vi "StartUp Sequence Open Loop Rev 1.4.vi"() -> ()   [LabVIEW 2017]
panel:
  in  "Set Pump Value 1":string
  out "Pump Value 2":string
  in  "Soft Shut Off":bool
  out "Pump Value 1":string
  in  "Send Pump":bool
  in  "Send Command":bool
  in  "Custom Command":string
  out "Startup Success":bool
  in  "Output File":path
  in  "Shut Off":bool
  out "ECU COM Port Out":refnum<visa-resource-name>
  out "Throttle Position":string
  out "Turbine RPM":string
  out "Turbine Temp":string
  out "Error Out":errorcluster
  in  "Error In":errorcluster
  in  "ECU COM Port":refnum<visa-resource-name>
  out "Turbine State":string
  in  "Strt Sqnc":bool
  # "Note: save to a .csv file"
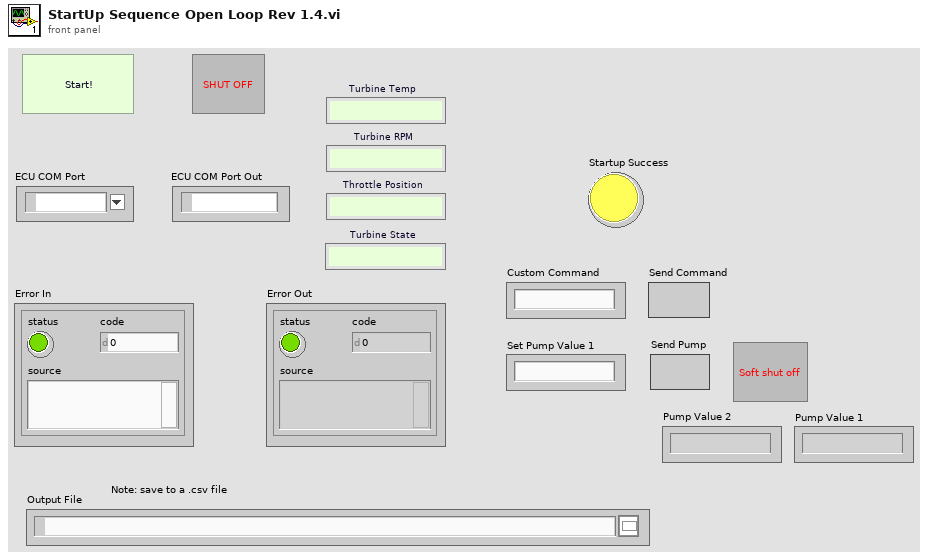
[diagram p1: front panel]
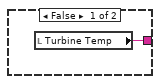
[diagram p4: hidden frame]
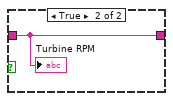
[diagram p5: hidden frame]
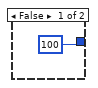
[diagram p7: hidden frame]
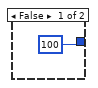
[diagram p8: hidden frame]
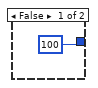
[diagram p9: hidden frame]
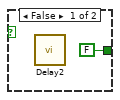
[diagram p11: hidden frame]
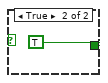
[diagram p12: hidden frame]
diagram:
  w7 = 21 ("Pulse Width")
  w8 = 160 ("Voltage")
  w13 = 16 ("Pulse Width")
  w14 = 160 ("Voltage")
  w4 = 255 ("y")
  w5 = 80 ("y")
  # "Disengage Starter Motor"
  # "Starter Motor 55%"
  # "Start button is inside a while loop that doesn't progess until True"
  # "Fuel Pump Mode 2"
  # "GlowPlugOff"
  # "Start Up\nFuelPumpMode 1"
  # "BurnerValveIgnitionPercent"
  # "If False, each Case structure is set\nto an arbitrary Delay time of 0.2 s"
  # "Each Stage is inside a while loop so that \nthe sequence doesn't progress until True"
  n1 = call "Initialize Com Port.vi"("Error In"="Error In", "ECU COM Port"="ECU COM Port") -> ("Error Out"=w28:errorcluster, "ECU COM Port Out"=w27:refnum<visa-resource-name>)  [unwired: 8 in]
  n2 = while {
    tunnel: w28 -> [w125]
    tunnel: [w125] -> w26
    stop <- "Strt Sqnc" stop-if-true
  }
  n3 = call "Initialize Output File.vi"("error in (no error)"=w26, "File Path Control"="Output File") -> ("error out"=w3:errorcluster)  [unwired: 9 in]
  n4 = flat-sequence {
    tunnel: w3 -> [w127]
    tunnel: [w127] -> w18
    frame #0 {
      n5 = local write "Strt Sqnc"(FALSE ("Strt Sqnc")) -> ()
    }
  }
  n6 = flat-sequence {
    tunnel: [w130] -> w2
    tunnel: w3 -> [w130]
    frame #0 {
      w129 = "0" ("Pump Value 1")
      n7 = local write "Pump Value 2"(w129) -> ()
      n8 = local write "Pump Value 1"(w129) -> ()
    }
  }
  n9 = while {
    tunnel: w2 -> [w148]
    tunnel: w27 -> [w147]
    tunnel: "Output File" -> [w144]
    stop <- w143 continue-if-true
    n10 = call "Get Engine Update.vi"("Error In"=w148, "ECU COM Port"=w147) -> ("Error Out"=w145:errorcluster, "Temperature"=w136:string, "RPMs"=w140:string, "ECU COM Port Out"=w142:refnum<visa-resource-name>)  [unwired: 6 in]
    n11 = call "Time Delay4"() -> ()  [unwired: 11 in, 1 out]
    n12 = call "Safety Check.vi"("Temperature"=w136, "RPMs"=w140) -> ("Safe?"=w143:bool)  [unwired: 9 in]
    n13 = Not Equal?(x=w140, y="") -> (x != y?=w138:bool)
    n14 = Not Equal?(x=w136, y="") -> (x != y?=w135:bool)
    n15 = case shown="False" w143 {
      selector: w143 -> [w153 w155]
      tunnel: w142 -> [w154 _]
      tunnel: [w153 w155] -> w141
      frame False {
        n16 = call "Emergency Shutoff.vi"("ECU COM Port"=w154) -> ()  [unwired: 9 in, 2 out]
      }
      frame True {
      }
    }
    n17 = case shown="False" w138 {
      tunnel: w140 -> [_ w152]
      tunnel: [w151 w152] -> w133
      frame False {
        n18 = local read "Turbine RPM"() -> (w151:string)
      }
      frame True {
        "Turbine RPM" <- w152
      }
    }
    n19 = case shown="True" w135 {
      tunnel: w136 -> [_ w150]
      tunnel: [w149 w150] -> w134
      frame False {
        n20 = local read "Turbine Temp"() -> (w149:string)
      }
      frame True {
        "Turbine Temp" <- w150
      }
    }
    n21 = Not(x=w141) -> (.not. x?=w146:bool)
    n22 = Stop(stop? (T)=w146) -> ()
    n23 = local read "Pump Value 2"() -> (w131:string)
    n24 = local read "Pump Value 1"() -> (w132:string)
    n25 = call "Write Data to Output File.vi"("Pump Value 2"=w131, "Pump Value 1"=w132, "Error In"=w145, "Temperature"=w134, "RPM"=w133, "File Path Control"=w144) -> ()  [unwired: 5 in, 1 out]
  }
  n26 = while {
    tunnel: w27 -> [w157]
    tunnel: w28 -> [_]
    stop <- FALSE stop-if-true
    n27 = case shown="True" "Send Command" {
      tunnel: "Custom Command" -> [_ w161]
      tunnel: w157 -> [_ w160]
      frame False {
      }
      frame True {
        n28 = call "Time Delay3"() -> ()  [unwired: 11 in, 1 out]
        n29 = VISA Write(VISA resource name=w160, write buffer=w161) -> ()  [unwired: 1 in, 3 out]
      }
    }
  }
  n30 = flat-sequence {
    tunnel: w18 -> [_]
    frame #0 {
      n31 = local write "Turbine State"("Initializing Motor") -> ()
    }
  }
  n32 = while {
    tunnel: ["Shut Off"] -> w122
    tunnel: "ECU COM Port" -> [w163]
    stop <- "Shut Off" stop-if-true
    # "Turns off each individual component"
    n33 = case shown="True" "Shut Off" {
      tunnel: w163 -> [_ w167]
      frame False {
      }
      frame True {
        n34 = call "Emergency Shutoff.vi"("ECU COM Port"=w167) -> ("Error Out"=w166:errorcluster)  [unwired: 9 in, 1 out]
        n35 = local write "Output File"(path "" ("Output File")) -> ()
        n36 = flat-sequence {
          tunnel: w166 -> [w168]
          tunnel: [w168] -> _
          frame #0 {
            n37 = local write "Strt Sqnc"(FALSE ("Strt Sqnc")) -> ()
          }
        }
      }
    }
  }
  n38 = call "Set Glow Plug Duty Cycle.vi"("Error In"=w18, "Duty Cycle"=6, "ECU COM Port"=w27) -> ("Error Out"=w113:errorcluster, "ECU COM Port Out"=w110:refnum<visa-resource-name>)  [unwired: 7 in]
  n39 = call "Delay"("error in (no error)"=w113) -> ("error out"=w112:errorcluster)  [unwired: 10 in]
  n40 = call "Set Glow Plug Duty Cycle.vi"("Error In"=w112, "Duty Cycle"=19, "ECU COM Port"=w110) -> ("Error Out"=w111:errorcluster, "ECU COM Port Out"=w106:refnum<visa-resource-name>)  [unwired: 7 in]
  n41 = call "Delay"("error in (no error)"=w111) -> ("error out"=w107:errorcluster)  [unwired: 10 in]
  n42 = call "Set Starter Motor Duty Cycle.vi"("Error In"=w107, "Duty Cycle"=6, "ECU COM Port"=w106) -> ("Error Out"=w105:errorcluster, "ECU COM Port Out"=w103:refnum<visa-resource-name>)  [unwired: 7 in]
  n43 = call "Set Glow Plug Duty Cycle.vi"("Error In"=w105, "Duty Cycle"=15, "ECU COM Port"=w103) -> ("Error Out"=w104:errorcluster, "ECU COM Port Out"=w99:refnum<visa-resource-name>)  [unwired: 7 in]
  n44 = call "Delay"("error in (no error)"=w104) -> ("error out"=w101:errorcluster)  [unwired: 10 in]
  n45 = call "Set Starter Motor Duty Cycle.vi"("Error In"=w101, "Duty Cycle"=4, "ECU COM Port"=w99) -> ("Error Out"=w100:errorcluster, "ECU COM Port Out"=w98:refnum<visa-resource-name>)  [unwired: 7 in]
  n46 = call "Delay"("error in (no error)"=w100) -> ("error out"=w123:errorcluster)  [unwired: 10 in]
  n47 = Stop(stop? (T)=w122) -> ()
  n48 = while {
    tunnel: w123 -> [w172]
    tunnel: w98 -> [w171]
    tunnel: [w171] -> w16
    tunnel: [w172] -> w124
    stop <- w175 stop-if-true
    n49 = local read "Turbine RPM"() -> (w170:string)
    n50 = Decimal String To Number(string=w170) -> (number=w174:i32)  [unwired: 2 in, 1 out]
    n51 = Greater Or Equal?(x=w174, y=3300) -> (x >= y?=w176:bool)
    n52 = case shown="True" w176 {
      tunnel: [FALSE TRUE] -> w175
      frame False {
        n53 = call "Delay2"() -> ()  [unwired: 11 in, 1 out]
      }
      frame True {
      }
    }
  }
  n54 = flat-sequence {
    tunnel: w123 -> [_]
    frame #0 {
      n55 = local write "Turbine State"("Stage1 Check RPM") -> ()
    }
  }
  n56 = call "CmdSeparator7"("error in (no error)"=w124) -> ("error out"=w12:errorcluster)  [unwired: 10 in]
  n57 = call "Set Pump Fow Rate.vi"("Error In"=w12, "Pulse Width"=w13, "Voltage"=w14, "ECU COM Port"=w16) -> ("Error Out"=w17:errorcluster, "ECU COM Port Out"=w15:refnum<visa-resource-name>)  [unwired: 6 in]
  n58 = flat-sequence {
    tunnel: w14 -> [w181]
    tunnel: w13 -> [w180]
    tunnel: w12 -> [_]
    frame #0 {
      n59 = Number To Decimal String(number=w180) -> (decimal integer string=w182:string)  [unwired: 1 in]
      n60 = Number To Decimal String(number=w181) -> (decimal integer string=w183:string)  [unwired: 1 in]
      n61 = local write "Pump Value 2"(w182) -> ()
      n62 = local write "Pump Value 1"(w183) -> ()
    }
  }
  n63 = call "CmdSeparator2"("error in (no error)"=w17) -> ("error out"=w97:errorcluster)  [unwired: 10 in]
  n64 = call "Set Burner Valve Percent.vi"("Error In"=w97, "Percent"=10, "ECU COM Port"=w15) -> ("Error Out"=w96:errorcluster, "ECU COM Port Out"=w86:refnum<visa-resource-name>)  [unwired: 7 in]
  n65 = call "CmdSeparator"("error in (no error)"=w96) -> ("error out"=w95:errorcluster)  [unwired: 10 in]
  n66 = call "Set Burner Valve Percent.vi"("Error In"=w95, "Percent"=31, "ECU COM Port"=w86) -> ("Error Out"=w94:errorcluster, "ECU COM Port Out"=w85:refnum<visa-resource-name>)  [unwired: 7 in]
  n67 = call "CmdSeparator10"("error in (no error)"=w94) -> ("error out"=w93:errorcluster)  [unwired: 10 in]
  n68 = call "Set Burner Valve Percent.vi"("Error In"=w93, "Percent"=35, "ECU COM Port"=w85) -> ("Error Out"=w92:errorcluster, "ECU COM Port Out"=w84:refnum<visa-resource-name>)  [unwired: 7 in]
  n69 = call "CmdSeparator11"("error in (no error)"=w92) -> ("error out"=w91:errorcluster)  [unwired: 10 in]
  n70 = call "Set Burner Valve Percent.vi"("Error In"=w91, "Percent"=39, "ECU COM Port"=w84) -> ("Error Out"=w90:errorcluster, "ECU COM Port Out"=w83:refnum<visa-resource-name>)  [unwired: 7 in]
  n71 = call "CmdSeparator12"("error in (no error)"=w90) -> ("error out"=w89:errorcluster)  [unwired: 10 in]
  n72 = call "Set Burner Valve Percent.vi"("Error In"=w89, "Percent"=43, "ECU COM Port"=w83) -> ("Error Out"=w88:errorcluster, "ECU COM Port Out"=w82:refnum<visa-resource-name>)  [unwired: 7 in]
  n73 = call "CmdSeparator13"("error in (no error)"=w88) -> ("error out"=w87:errorcluster)  [unwired: 10 in]
  n74 = call "Set Burner Valve Percent.vi"("Error In"=w87, "Percent"=47, "ECU COM Port"=w82) -> ("Error Out"=w65:errorcluster, "ECU COM Port Out"=w64:refnum<visa-resource-name>)  [unwired: 7 in]
  n75 = call "CmdSeparator6"("error in (no error)"=w65) -> ("error out"=w67:errorcluster)  [unwired: 10 in]
  n76 = call "Set Burner Valve Percent.vi"("Error In"=w67, "Percent"=51, "ECU COM Port"=w64) -> ("Error Out"=w60:errorcluster, "ECU COM Port Out"=w61:refnum<visa-resource-name>)  [unwired: 7 in]
  n77 = call "CmdSeparator8"("error in (no error)"=w60) -> ("error out"=w63:errorcluster)  [unwired: 10 in]
  n78 = call "Set Burner Valve Percent.vi"("Error In"=w63, "Percent"=55, "ECU COM Port"=w61) -> ("Error Out"=w56:errorcluster, "ECU COM Port Out"=w57:refnum<visa-resource-name>)  [unwired: 7 in]
  n79 = call "CmdSeparator14"("error in (no error)"=w56) -> ("error out"=w59:errorcluster)  [unwired: 10 in]
  n80 = call "Set Burner Valve Percent.vi"("Error In"=w59, "Percent"=59, "ECU COM Port"=w57) -> ("Error Out"=w55:errorcluster, "ECU COM Port Out"=w54:refnum<visa-resource-name>)  [unwired: 7 in]
  n81 = call "CmdSeparator9"("error in (no error)"=w55) -> ("error out"=w121:errorcluster)  [unwired: 10 in]
  n82 = flat-sequence {
    tunnel: w121 -> [_]
    frame #0 {
      n83 = local write "Turbine State"("Stage2 Check Temp.") -> ()
    }
  }
  n84 = while {
    tunnel: w54 -> [w186]
    tunnel: w121 -> [w187]
    tunnel: [w186] -> w71
    tunnel: [w187] -> w72
    stop <- w190 stop-if-true
    # "Stage2Temp(C)"
    n85 = local read "Turbine Temp"() -> (w185:string)
    n86 = Decimal String To Number(string=w185) -> (number=w188:i32)  [unwired: 2 in, 1 out]
    n87 = Greater Or Equal?(x=w188, y=90) -> (x >= y?=w191:bool)
    n88 = case shown="False" w191 {
      tunnel: [FALSE TRUE] -> w190
      frame False {
        n89 = call "Delay3"() -> ()  [unwired: 11 in, 1 out]
      }
      frame True {
      }
    }
  }
  n90 = call "Set Glow Plug Duty Cycle.vi"("Error In"=w72, "Duty Cycle"=0, "ECU COM Port"=w71) -> ("Error Out"=w70:errorcluster, "ECU COM Port Out"=w9:refnum<visa-resource-name>)  [unwired: 7 in]
  n91 = call "CmdSeparator3"("error in (no error)"=w70) -> ("error out"=w6:errorcluster)  [unwired: 10 in]
  n92 = call "Set Pump Fow Rate.vi"("Error In"=w6, "Pulse Width"=w7, "Voltage"=w8, "ECU COM Port"=w9) -> ("Error Out"=w11:errorcluster, "ECU COM Port Out"=w10:refnum<visa-resource-name>)  [unwired: 6 in]
  n93 = call "Set Burner Valve Percent.vi"("Error In"=w11, "Percent"=80, "ECU COM Port"=w10) -> ("Error Out"=w53:errorcluster, "ECU COM Port Out"=w68:refnum<visa-resource-name>)  [unwired: 7 in]
  n94 = flat-sequence {
    tunnel: w8 -> [w195]
    tunnel: w7 -> [w194]
    tunnel: w6 -> [_]
    frame #0 {
      n95 = Number To Decimal String(number=w194) -> (decimal integer string=w196:string)  [unwired: 1 in]
      n96 = Number To Decimal String(number=w195) -> (decimal integer string=w197:string)  [unwired: 1 in]
      n97 = local write "Pump Value 2"(w196) -> ()
      n98 = local write "Pump Value 1"(w197) -> ()
    }
  }
  n99 = call "CmdSeparator18"("error in (no error)"=w53) -> ("error out"=w52:errorcluster)  [unwired: 10 in]
  n100 = call "Set Fuel Valve Percent.vi"("Error In"=w52, "Percent"=12, "ECU COM Port"=w68) -> ("Error Out"=w51:errorcluster, "ECU COM Port Out"=w69:refnum<visa-resource-name>)  [unwired: 7 in]
  n101 = call "CmdSeparator16"("error in (no error)"=w51) -> ("error out"=w119:errorcluster)  [unwired: 10 in]
  n102 = for {
    N: 4 -> [_]
    tunnel: [w198] -> _
    tunnel: [w212] -> _
    tunnel: w69 -> [w204]
    tunnel: w119 -> [w205]
    shift-right: [w203] -> w47
    shift-left: 12 -> [w209]
    shift-right: [w200] -> _
    shift-left: 80 -> [w206]
    tunnel: [w212] -> w42 mode=indexing
    tunnel: [w198] -> w48 mode=indexing
    n103 = Less?(x=w209, y=100) -> (x < y?=w210:bool)
    n104 = Less?(x=w206, y=100) -> (x < y?=w207:bool)
    n105 = case shown="True" w207 {
      tunnel: w206 -> [_ w216]
      tunnel: [100 w214] -> w200
      frame False {
      }
      frame True {
        n106 = Add(x=w216, y=5) -> (x+y=w214:i32)
      }
    }
    n107 = case shown="True" w210 {
      tunnel: w209 -> [_ w220]
      tunnel: [100 w218] -> w203
      frame False {
      }
      frame True {
        n108 = Add(x=w220, y=6) -> (x+y=w218:i32)
      }
    }
    n109 = call "Set Fuel Valve Percent.vi"("Error In"=w205, "Percent"=w203, "ECU COM Port"=w204) -> ("Error Out"=w202:errorcluster, "ECU COM Port Out"=w199:refnum<visa-resource-name>)  [unwired: 7 in]
    n110 = call "Set Burner Valve Percent.vi"("Error In"=w202, "Percent"=w200, "ECU COM Port"=w199) -> ("Error Out"=w201:errorcluster, "ECU COM Port Out"=w198:refnum<visa-resource-name>)  [unwired: 7 in]
    n111 = call "CmdSeparator17"("error in (no error)"=w201) -> ("error out"=w212:errorcluster)  [unwired: 10 in]
  }
  n112 = flat-sequence {
    tunnel: w42 -> [_]
    frame #0 {
      n113 = local write "Turbine State"("Pump Ramp Up") -> ()
    }
  }
  n114 = for {
    N: 10 -> [_]
    tunnel: [w228] -> w30
    tunnel: [w239] -> w33
    shift-right: [w235] -> _
    shift-left: w47 -> [w236]
    tunnel: w42 -> [w232] mode=indexing
    tunnel: w48 -> [w231] mode=indexing
    shift-right: [w224] -> w44
    shift-left: 21 -> [w225]
    w223 = 160 ("y")
    n115 = Less?(x=w236, y=100) -> (x < y?=w237:bool)
    n116 = Add(x=w225, y=1) -> (x+y=w224:i32)
    n117 = case shown="True" w237 {
      tunnel: w236 -> [_ w247]
      tunnel: [100 w245] -> w235
      frame False {
      }
      frame True {
        n118 = Add(x=w247, y=5) -> (x+y=w245:i32)
      }
    }
    n119 = call "Set Fuel Valve Percent.vi"("Error In"=w232, "Percent"=w235, "ECU COM Port"=w231) -> ("Error Out"=w234:errorcluster, "ECU COM Port Out"=w233:refnum<visa-resource-name>)  [unwired: 7 in]
    n120 = call "Set Burner Valve Percent.vi"("Error In"=w234, "Percent"=100 ("y"), "ECU COM Port"=w233) -> ("Error Out"=w222:errorcluster, "ECU COM Port Out"=w229:refnum<visa-resource-name>)  [unwired: 7 in]
    n121 = call "Set Pump Fow Rate.vi"("Error In"=w222, "Pulse Width"=w224, "Voltage"=w223, "ECU COM Port"=w229) -> ("Error Out"=w227:errorcluster, "ECU COM Port Out"=w228:refnum<visa-resource-name>)  [unwired: 6 in]
    n122 = flat-sequence {
      tunnel: w223 -> [w241]
      tunnel: w224 -> [w240]
      tunnel: w222 -> [_]
      frame #0 {
        n123 = Number To Decimal String(number=w240) -> (decimal integer string=w242:string)  [unwired: 1 in]
        n124 = Number To Decimal String(number=w241) -> (decimal integer string=w243:string)  [unwired: 1 in]
        n125 = local write "Pump Value 2"(w242) -> ()
        n126 = local write "Pump Value 1"(w243) -> ()
      }
    }
    n127 = call "CmdSeparator20"("error in (no error)"=w227) -> ("error out"=w239:errorcluster)  [unwired: 10 in]
  }
  n128 = call "Set Starter Motor Duty Cycle.vi"("Error In"=w33, "Duty Cycle"=11, "ECU COM Port"=w30) -> ("Error Out"=w32:errorcluster, "ECU COM Port Out"=w31:refnum<visa-resource-name>)  [unwired: 7 in]
  n129 = flat-sequence {
    tunnel: w32 -> [_]
    frame #0 {
      n130 = local write "Turbine State"("Secondary Pump Ramp Up") -> ()
    }
  }
  n131 = for {
    N: 3 -> [_]
    tunnel: [w256] -> w43
    tunnel: [w263] -> w41
    tunnel: w32 -> [w260]
    tunnel: w31 -> [w259]
    shift-right: [w250] -> _
    shift-left: w44 -> [w253]
    w251 = 160 ("y")
    n132 = Add(x=w253, y=10) -> (x+y=w250:i32)
    n133 = call "Set Fuel Valve Percent.vi"("Error In"=w260, "Percent"=100 ("y"), "ECU COM Port"=w259) -> ("Error Out"=w262:errorcluster, "ECU COM Port Out"=w261:refnum<visa-resource-name>)  [unwired: 7 in]
    n134 = call "Set Burner Valve Percent.vi"("Error In"=w262, "Percent"=0 ("y"), "ECU COM Port"=w261) -> ("Error Out"=w249:errorcluster, "ECU COM Port Out"=w257:refnum<visa-resource-name>)  [unwired: 7 in]
    n135 = call "Set Pump Fow Rate.vi"("Error In"=w249, "Pulse Width"=w250, "Voltage"=w251, "ECU COM Port"=w257) -> ("Error Out"=w255:errorcluster, "ECU COM Port Out"=w256:refnum<visa-resource-name>)  [unwired: 6 in]
    n136 = flat-sequence {
      tunnel: w251 -> [w265]
      tunnel: w250 -> [w264]
      tunnel: w249 -> [_]
      frame #0 {
        n137 = Number To Decimal String(number=w264) -> (decimal integer string=w266:string)  [unwired: 1 in]
        n138 = Number To Decimal String(number=w265) -> (decimal integer string=w267:string)  [unwired: 1 in]
        n139 = local write "Pump Value 2"(w266) -> ()
        n140 = local write "Pump Value 1"(w267) -> ()
      }
    }
    n141 = call "CmdSeparator15"("error in (no error)"=w255) -> ("error out"=w263:errorcluster)  [unwired: 10 in]
  }
  n142 = flat-sequence {
    tunnel: w41 -> [_]
    frame #0 {
      n143 = local write "Turbine State"("Hold on to your butts!") -> ()
    }
  }
  n144 = while {
    tunnel: w41 -> [w270]
    tunnel: w43 -> [w269]
    tunnel: [w270] -> w1
    tunnel: [w269] -> w40
    stop <- w271 stop-if-true
    n145 = local read "Turbine RPM"() -> (w274:string)
    n146 = Decimal String To Number(string=w274) -> (number=w273:i32)  [unwired: 2 in, 1 out]
    n147 = Greater?(x=w273, y=30000) -> (0:w271:bool)
  }
  n148 = call "Set Pump Fow Rate.vi"("Error In"=w1, "Pulse Width"=w4, "Voltage"=w5, "ECU COM Port"=w40) -> ("Error Out"=w39:errorcluster, "ECU COM Port Out"=w38:refnum<visa-resource-name>)  [unwired: 6 in]
  n149 = flat-sequence {
    tunnel: w5 -> [w277]
    tunnel: w4 -> [w276]
    tunnel: [w275] -> _
    tunnel: w1 -> [w275]
    frame #0 {
      n150 = Number To Decimal String(number=w276) -> (decimal integer string=w278:string)  [unwired: 1 in]
      n151 = Number To Decimal String(number=w277) -> (decimal integer string=w279:string)  [unwired: 1 in]
      n152 = local write "Pump Value 2"(w278) -> ()
      n153 = local write "Pump Value 1"(w279) -> ()
    }
  }
  n154 = while {
    tunnel: w39 -> [w281]
    tunnel: w38 -> [w280]
    tunnel: [w281] -> w35
    tunnel: [w280] -> w37
    stop <- w282 stop-if-true
    n155 = local read "Turbine RPM"() -> (w285:string)
    n156 = Decimal String To Number(string=w285) -> (number=w284:i32)  [unwired: 2 in, 1 out]
    n157 = Greater?(x=w284, y=44000) -> (0:w282:bool)
  }
  n158 = flat-sequence {
    tunnel: w35 -> [_]
    frame #0 {
      n159 = local write "Turbine State"("Acheived Idle RPM!") -> ()
    }
  }
  n160 = call "Set Starter Motor Duty Cycle.vi"("Error In"=w35, "Duty Cycle"=0, "ECU COM Port"=w37) -> ("Error Out"=w24:errorcluster, "ECU COM Port Out"=w23:refnum<visa-resource-name>)  [unwired: 7 in]
  n161 = flat-sequence {
    tunnel: w24 -> [_]
    frame #0 {
      "Startup Success" <- TRUE
    }
  }
  n162 = while {
    tunnel: w23 -> [w300]
    tunnel: [w299] -> w21
    tunnel: [w298] -> w22
    tunnel: w24 -> [w296]
    stop <- "Soft Shut Off" stop-if-true
    n163 = Decimal String To Number(string="Set Pump Value 1") -> (number=w297:i32)  [unwired: 2 in, 1 out]
    n164 = Less?(x=w297, y=255) -> (x < y?=w292:bool)
    n165 = Greater Than 0?(x=w297) -> (x > 0?=w293:bool)
    n166 = And(x=w293, y=w292) -> (x .and. y?=w290:bool)
    n167 = call "Time Delay"() -> ()  [unwired: 11 in, 1 out]
    n168 = And(x=w290, y="Send Pump") -> (x .and. y?=w288:bool)
    n169 = case shown="True" w288 {
      tunnel: w300 -> [w301 w310]
      tunnel: w296 -> [w302 w309]
      tunnel: [w301 w308] -> w299
      tunnel: [w302 w307] -> w298
      tunnel: w297 -> [_ w304]
      frame False {
      }
      frame True {
        n170 = call "Set Pump Fow Rate.vi"("Error In"=w309, "Pulse Width"=255, "Voltage"=w304, "ECU COM Port"=w310) -> ("Error Out"=w307:errorcluster, "ECU COM Port Out"=w308:refnum<visa-resource-name>)  [unwired: 6 in]
        n171 = Number To Decimal String(number=w304) -> (decimal integer string=→"Pump Value 1":string)  [unwired: 1 in]
        n172 = local write "Pump Value 2"("255" ("Pump Value 2")) -> ()
      }
    }
  }
  n173 = call "Emergency Shutoff.vi"("Error In"=w22, "ECU COM Port"=w21) -> ("Error Out"=w20:errorcluster, "ECU COM Port Out"=→"ECU COM Port Out":refnum<visa-resource-name>)  [unwired: 8 in]
  n174 = flat-sequence {
    tunnel: w20 -> [w311]
    tunnel: [w311] -> w120
    frame #0 {
    }
  }
  "Error Out" <- w120
